vi "Configure.vi"(8 "error in (no error)":errorcluster, 10 "ID":string, 11 "MKS901P in":refnum<class "MKS901P.lvclass">) -> (0 "error out":errorcluster, 3 "MKS901P out":refnum<class "MKS901P.lvclass">)   [LabVIEW 2016, in "MKS901P.lvlib" / "MKS901P.lvclass"]
uses:
  MKS901P.lvclass
  MKS901P.lvclass/MKS901P.ctl
  <vilib>/Utility/config.llb/Read Key (U32).vi
  <vilib>/Utility/config.llb/Read Key (String).vi
  <vilib>/Utility/config.llb/NI_LVConfig.lvlib
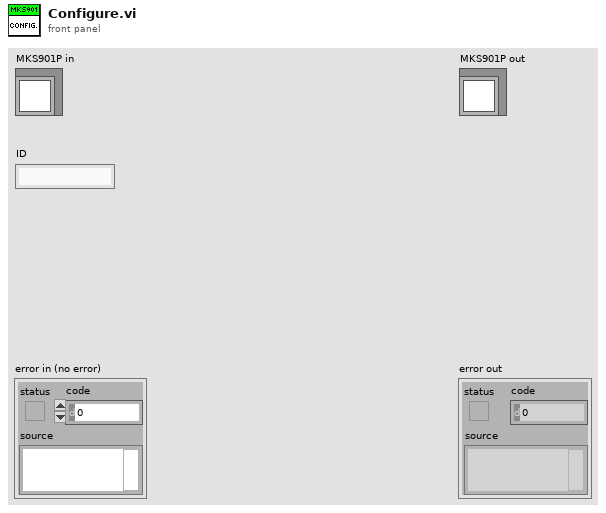
[diagram p1: front panel]
types:
  T1 = typedef "NI_LVConfig.lvlib/Config Data RefNum.ctl" = refnum<k1>
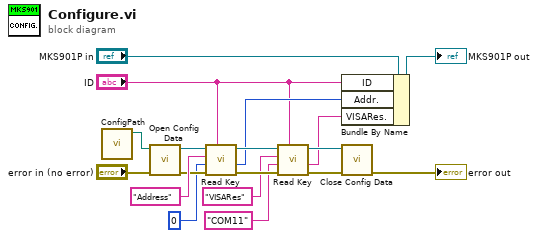
[diagram p0: block diagram]
diagram:
  n1 = call "ConfigPath.vi"() -> ("ConfigPath"=w18:path)  [unwired: 11 in]
  n2 = call <vilib>:"Open Config Data.vi"("error in (no error)"="error in (no error)", "configuration file path"=w18) -> ("error out"=w15:errorcluster, "refnum"=w17:T1)  [unwired: 7 in, 1 out]
  n3 = call-poly <vilib>:"Read Key.vi"("section"="ID", "error in (no error)"=w15, "default value"=u8 0, "key"="Address", "refnum"=w17) -> ("error out"=w13:errorcluster, "value"=w9:u32, "refnum out"=w14:T1)  [unwired: 3 in, 1 out]
  n4 = call-poly <vilib>:"Read Key.vi"("section"="ID", "error in (no error)"=w13, "default value"="COM11" ("key"), "key"="VISARes", "refnum"=w14) -> ("error out"=w11:errorcluster, "value"=w6:string, "refnum out"=w12:T1)  [unwired: 3 in, 1 out]
  n5 = Bundle By Name(cluster="MKS901P in", "ID"="ID", "Addr."=w9, "VISARes."=w6) -> (→"MKS901P out":refnum<class "MKS901P.lvclass">)
  n6 = call <vilib>:"Close Config Data.vi"("error in (no error)"=w11, "refnum"=w12) -> ("error out"=→"error out":errorcluster)  [unwired: 8 in, 1 out]
